vi "Configure.vi"(8 "error in (no error)":errorcluster, 11 "Camera_Prime95B in":refnum<class "Camera_Prime95B.lvclass">) -> (0 "error out":errorcluster, 3 "Camera_Prime95B out":refnum<class "Camera_Prime95B.lvclass">)   [LabVIEW 2020, in "Camera_Prime95B.lvlib" / "Camera_Prime95B.lvclass"]
uses:
  Camera_Prime95B.lvclass
  <vilib>/vision/Image Controls.llb/IMAQ Image.ctl
  Camera_Prime95B.lvclass/Camera_Prime95B.ctl
  E:/Development/DevHardSoftware/MMicroscopyAF/Model/Real Hardware/Camera_Prime95B/Camera_Prime95B/Dependencies/PVCamNET.dll
  Dependencies/PVCamNET.dll
  HAL Layer/Camera/Camera/Camera.lvclass
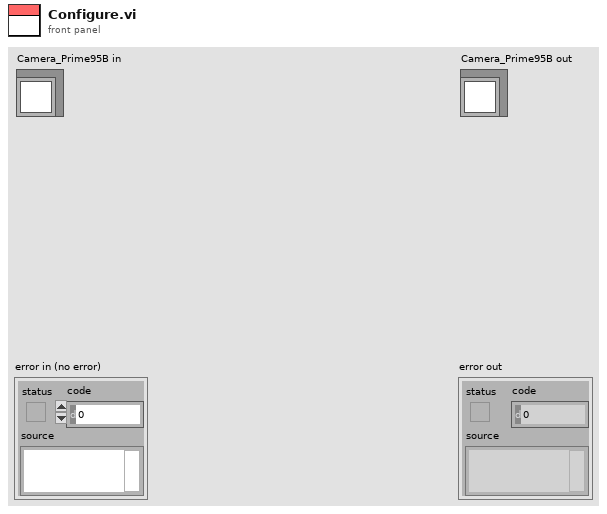
[diagram p1: front panel]
types:
  T1 = typedef "IMAQ Image.ctl" = refnum<image>
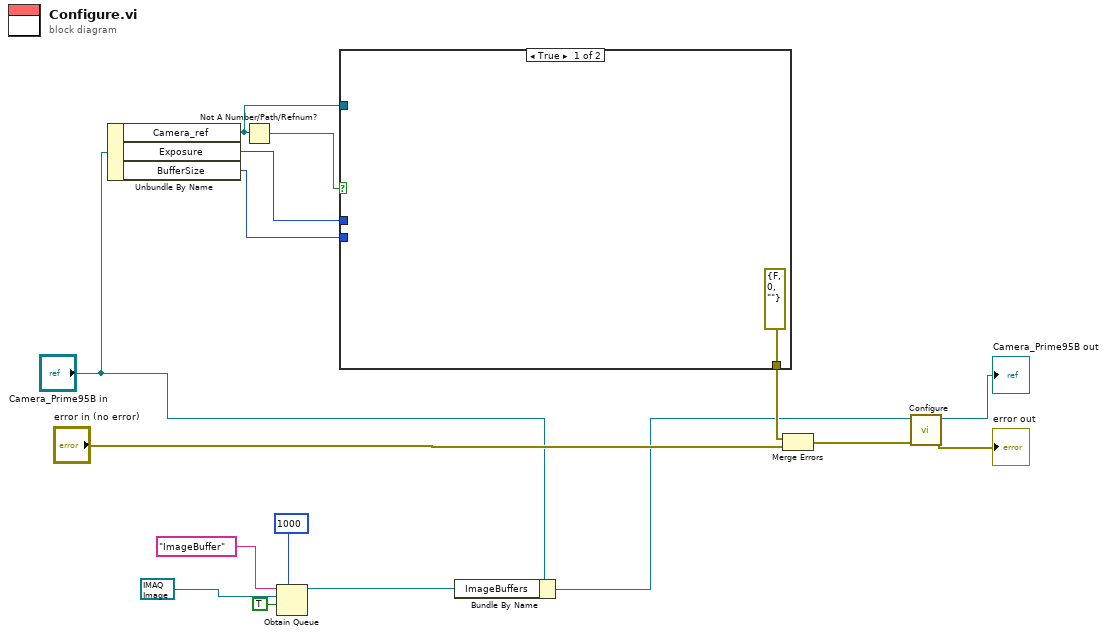
[diagram p0: block diagram]
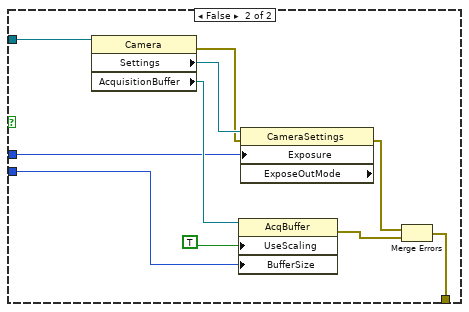
[diagram p2: hidden frame]
diagram:
  n1 = Unbundle By Name("Camera_Prime95B in") -> ("Camera_ref"=w14:refnum<k24>, "Exposure"=w11:i32, "BufferSize"=w12:i32)
  n2 = Not A Number/Path/Refnum?(number/path/refnum=w14) -> (NaN/Path/Refnum?=w13:bool)
  n3 = Obtain Queue(max queue size (-1, unlimited)=1000, name (unnamed)="ImageBuffer", element data type=T1 refnum ("New Image"), create if not found? (T)=TRUE) -> (queue out=w1:refnum<queue>)  [unwired: 1 in, 2 out]
  n4 = case shown="True" w13 {
    tunnel: w14 -> [_ w27]
    tunnel: w12 -> [_ w23]
    tunnel: w11 -> [_ w22]
    tunnel: [errorcluster {"status"=FALSE, "code"=0, "source"=""} ("error IO") w18] -> w8
    frame True {
    }
    frame False {
      n5 = property class="Camera"(reference=w27) -> (error out=w21:errorcluster, "Settings"=w26:refnum<k24>, "AcquisitionBuffer"=w25:refnum<k24>)  [unwired: 1 in, 1 out]
      n6 = property class="AcqBuffer"(reference=w25, "UseScaling"=TRUE, "BufferSize"=w23) -> (error out=w19:errorcluster)  [unwired: 1 in, 1 out]
      n7 = property class="CameraSettings" props=["Exposure", "ExposeOutMode"](reference=w26, error in=w21, "Exposure"=w22) -> (error out=w20:errorcluster)  [unwired: 2 out]
      n8 = Merge Errors(w20, w19) -> (w18:errorcluster)
    }
  }
  n9 = Bundle By Name(cluster="Camera_Prime95B in", "ImageBuffers"=w1) -> (w2:refnum<class "Camera_Prime95B.lvclass">)
  n10 = Merge Errors(w8, "error in (no error)") -> (w9:errorcluster)
  n11 = call-parent "Configure.vi"("error in (no error)"=w9, "Device in"=w2) -> ("error out"=→"error out":errorcluster, "Device out"=→"Camera_Prime95B out":refnum<class "Camera_Prime95B.lvclass">)  [unwired: 8 in]
